vi "Calculate farfield intensity.vi"(1 "h_pSLM":u8[][](array[numeric]), 2 "Numeric":i32=512) -> (0 "Calculated image plane":dbl[][](array[numeric]))   [LabVIEW 2009]
uses:
  <vilib>/Analysis/2dsp.llb/2D Inverse Complex FFT.vi
  <vilib>/Analysis/NI_AALPro.lvlib
panel:
  out "calculated image plane":dbl[][](graph)
  out "Displayed Hologram":u8[][](graph)
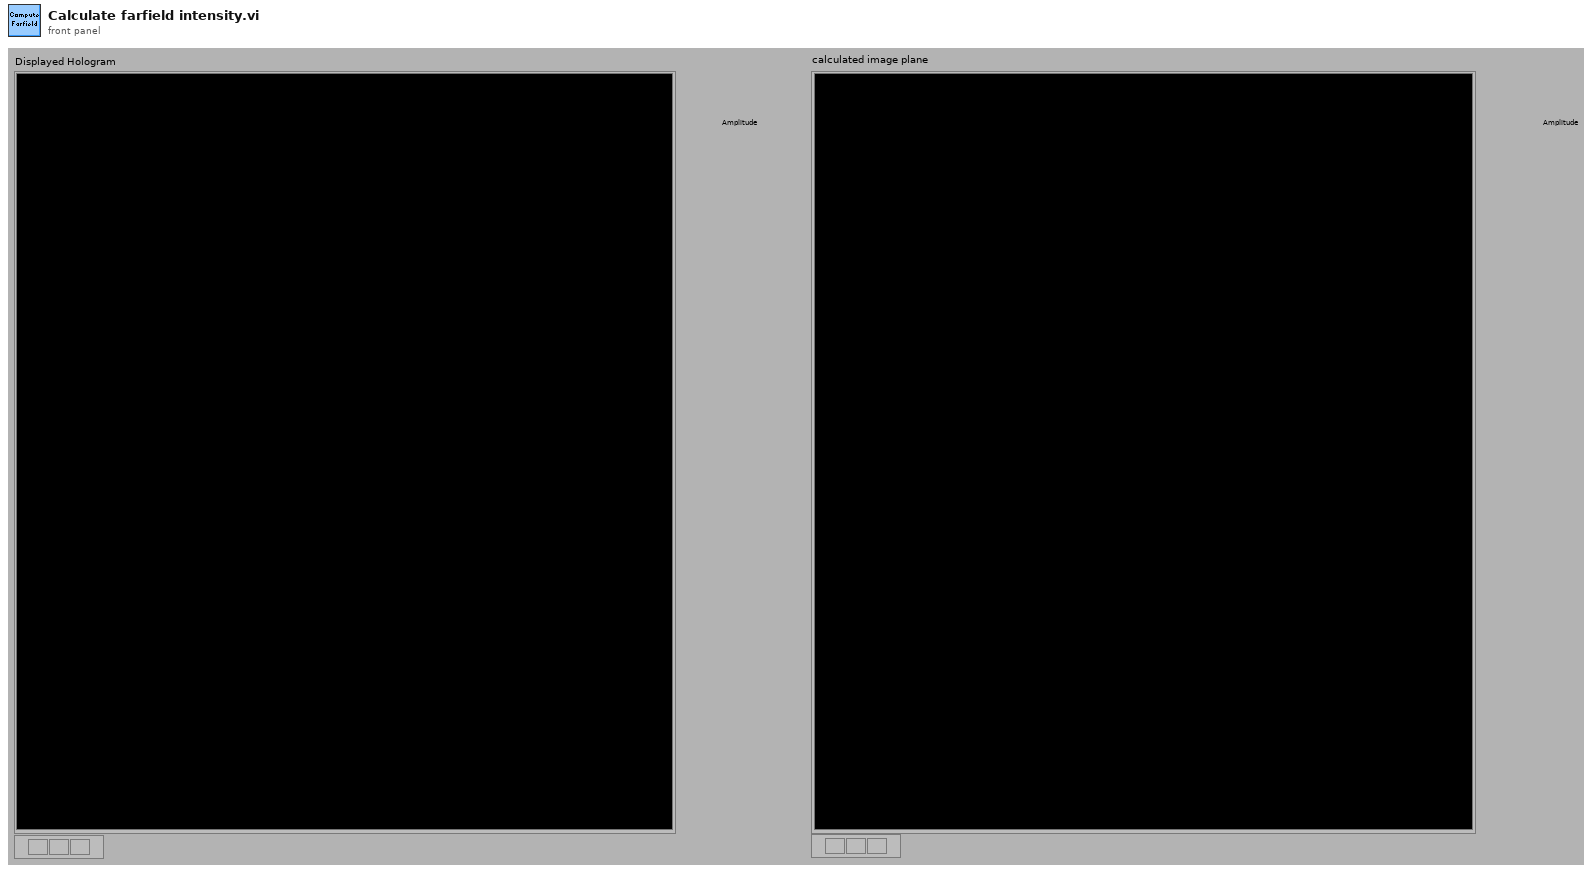
[diagram p1: front panel]
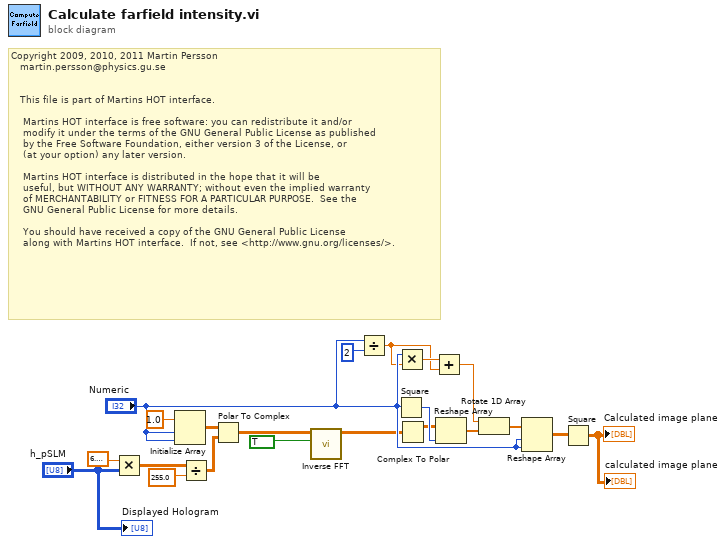
[diagram p0: block diagram]
diagram:
  # "Copyright 2009, 2010, 2011 Martin Persson \n   martin.persson@physics.gu.se\n\n\n   This file is part of Martins HOT interface.\n\n    Martins HOT interface is free software: you can redistribute it and/or \n    modify it under the terms of the GNU General Public License as published \n    by the Free Software Foundation, either version 3 of the License, or\n    (at your option) any later version.\n\n    Martins HOT interface is distributed in the hope that it will be \n    useful, but WITHOUT ANY WARRANTY; without even the implied warranty\n    of MERCHANTABILITY or FITNESS FOR A PARTICULAR PURPOSE.  See the\n    GNU General Public License for more details.\n\n    You should have received a copy of the GNU General Public License\n    along with Martins HOT interface.  If not, see <http://www.gnu.org/licenses/>."
  n1 = Multiply(x=6.283185307179586, y="h_pSLM") -> (x*y=w7:dbl[][])
  n2 = Initialize Array(1.0 ("element"), "Numeric", "Numeric") -> (w10:dbl[][])
  n3 = Divide(x=w7, y=255.0) -> (x/y=w9:dbl[][])
  n4 = Polar To Complex(1:w9, 2:w10) -> (0:w8:cdb[][])
  n5 = call-poly <vilib>:"Inverse FFT.vi"("shift?"=TRUE, "FFT {x}"=w8) -> ("X"=w5:cdb[][])  [unwired: 8 in, 1 out]
  n6 = Divide(x="Numeric", y=2) -> (x/y=w16:dbl)
  n7 = Square(x="Numeric") -> (x^2=w13:i32)
  n8 = Multiply(x="Numeric", y=w16) -> (x*y=w17:dbl)
  n9 = Complex To Polar(r * e^(i*theta)=w5) -> (r=w12:dbl[][])  [unwired: 1 out]
  n10 = Add(x=w17, y=w16) -> (x+y=w18:dbl)
  n11 = Reshape Array(w12, w13) -> (w14:dbl[])
  n12 = Rotate 1D Array(1:w14, 2:w18) -> (0:w19:dbl[])
  n13 = Reshape Array(w19, "Numeric", "Numeric") -> (w21:dbl[][])
  n14 = Square(x=w21) -> (x^2=→"Calculated image plane" →"calculated image plane":dbl[][])
  "Displayed Hologram" <- "h_pSLM"
